vi "Drivetrain Loop.vi"   [LabVIEW 2014]
uses:
  Robot Global Data.vi
  <vilib>/Rock Robotics/WPI/RobotDrive/WPI_RobotDriveArcadeDrive_Standard(NoSaturation).vi
  Common Code/Change Detect Double.vi
types:
  T1 = typedef "WPI_RobotDriveDevRef.ctl" = cluster{"DevStatus":errorcluster, "Motors[]":T2[], "Square Inputs":bool, "Max Output":dbl}
  T2 = typedef "WPI_MotorControlDeviceRef.ctl" = cluster{"DeviceStatus":errorcluster, "Type":T3, "PWM":cluster{"Controller":T4, "PWM Channel":T5, "DeadBand":T6}, "CAN":cluster{"Device Number":u8, "Control Mode":T7, "Semaphore":T8, "Max Vout":dbl, "TalonSRX Control Mode":T9}, "Invert":bool, "TransformRef":T10, "InvTransformRef":T10}
  T3 = typedef "WPI_MotorControlType.ctl" = enum16{"PWM", "CAN", "CANTalonSRX"}
  T4 = typedef "FPGA_TypedefDigitalModule.ctl" = enum16{"Controller 1"}
  T5 = typedef "FPGA_DIOPWMChannel.ctl" = enum8{"PWM 0", "PWM 1", "PWM 2", "PWM 3", "PWM 4", "PWM 5", "PWM 6", "PWM 7", "PWM 8", "PWM 9", "PWM MXP 0", "PWM MXP 1", "PWM MXP 2", "PWM MXP 3", "PWM MXP 4", "PWM MXP 5", "PWM MXP 6", "PWM MXP 7", "PWM MXP 8", "PWM MXP 9", "Invalid"}
  T6 = typedef "WPI_PWMDeadband.ctl" = cluster{"Name":string, "maxPositivePwm":i32, "minPositivePwm":i32, "centerPwm":i32, "maxNegativePwm":i32, "minNegativePwm":i32, "angularRange":u16}
  T7 = typedef "WPI_CANJaguar_ControlMode.ctl" = enum8{"Percent VBus", "Current", "Speed", "Position", "Voltage"}
  T8 = typedef "Semaphore RefNum" = refnum<k1>
  T9 = typedef "WPI_CANTalonSRX_APIControlMode.ctl" = enum8{"Percent VBus", "Speed", "Position", "Slave", "Unchanged / Invalid"}
  T10 = typedef "WPI_PWMTransform_ConPane.ctl" = refnum<vi>
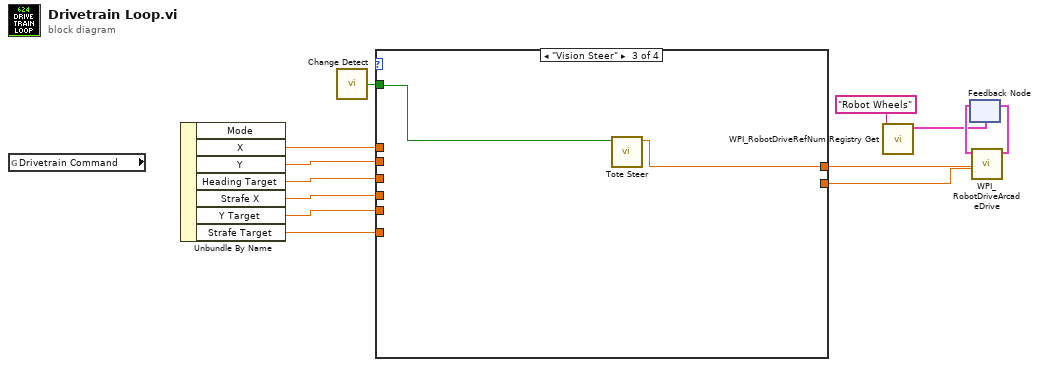
[diagram p0: block diagram]
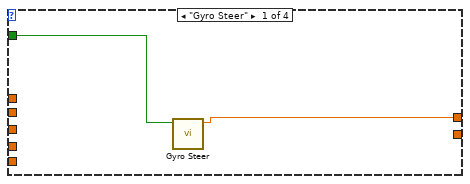
[diagram p2: hidden frame]
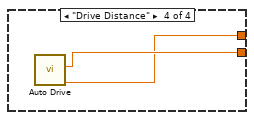
[diagram p4: hidden frame]
diagram:
  n1 = global read "Robot Global Data.vi" "Drivetrain Command"() -> ()  [unwired: 1 out]
  n2 = Unbundle By Name() -> ("X"=w4:dbl, "Y"=w7:dbl, "Heading Target"=w6:dbl, "Strafe X"=w3:dbl, "Y Target"=w2:dbl, "Strafe Target"=w1:dbl)  [unwired: 1 in, 1 out]
  n3 = call-poly "Change Detect.vi"() -> ("Changed?"=w5:bool)  [unwired: 1 in]
  n4 = case shown="\"Vision Steer\"" {
    selector: _ -> [_ _ _ _]
    tunnel: [w15 _ w17 w19] -> w9
    tunnel: w4 -> [_ _ _ _]
    tunnel: [_ _ _ w20] -> w8
    tunnel: w7 -> [_ _ _ _]
    tunnel: w6 -> [_ _ _ _]
    tunnel: w5 -> [w14 _ w16 _]
    tunnel: w3 -> [_ _ _ _]
    tunnel: w2 -> [_ _ _ _]
    tunnel: w1 -> [_ _ _ _]
    frame "Gyro Steer" {
      n5 = call "Gyro Steer.vi"("Changed?"=w14) -> ("X out"=w15:dbl)  [unwired: 10 in]
    }
    frame "Manual", Default {
    }
    frame "Vision Steer" {
      n6 = call "Tote Steer.vi"("Changed?"=w16) -> ("f"=w17:dbl)  [unwired: 10 in]
    }
    frame "Drive Distance" {
      n7 = call "Auto Drive.vi"() -> ("X out"=w19:dbl, "Strafe out"=w18:dbl, "Y out"=w20:dbl)  [unwired: 9 in]
    }
  }
  n8 = call <vilib>:"WPI_RobotDriveRefNum Registry Get.vi"("refnum name"="Robot Wheels") -> ("RobotDriveDevRef"=w10:T1)  [unwired: 9 in, 1 out]
  n9 = feedback #1(w10) -> (w11:T1)
  n10 = call-poly <vilib>:"WPI_RobotDriveArcadeDrive.vi"("Y axis value"=w8, "X axis value"=w9, "RobotDriveDevRef"=w11) -> ("RobotDriveDevRef"=w12:T1)  [unwired: 6 in, 2 out]
  n11 = feedback-in #1(w12) -> ()
